vi "Save Asset.vi"(8 "Error In":errorcluster, 11 "Asset":refnum<class "Asset.lvclass">) -> (0 "Error Out":errorcluster)   [LabVIEW 2019, in "Asset.lvclass"]
doc: "Save an asset for ingestion into the Asset Management service."
uses:
  Asset.lvclass
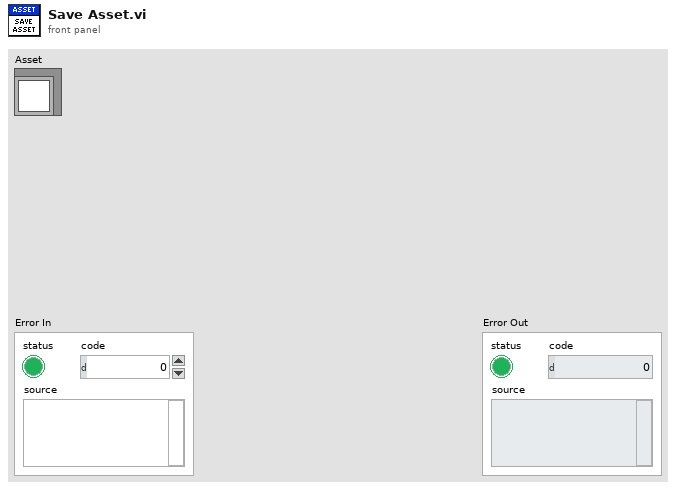
[diagram p1: front panel]
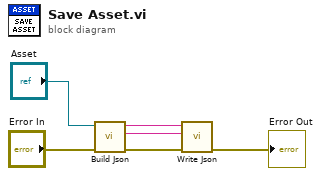
[diagram p0: block diagram]
diagram:
  n1 = call "Build Json.vi"("Error In"="Error In", "Asset"="Asset") -> ("Error Out"=w2:errorcluster, "JSON File Content"=w3:string, "JSON File Name"=w4:string)  [unwired: 7 in]
  n2 = call "Write Json.vi"("Error In"=w2, "JSON File Content"=w3, "JSON File Name"=w4) -> ("Error Out"=→"Error Out":errorcluster)  [unwired: 8 in]
